vi "day 19 task 1.vi"   [LabVIEW 2019]
uses:
  day 19/robot quantity at time--cluster.ctl
  day 19/supplies--cluster.ctl
  day 19/blueprint--cluster.ctl
types:
  T1 = typedef "supplies--cluster.ctl" = cluster{"ore":i32, "clay":i32, "obsidian":i32, "geode":i32}
  T2 = typedef "robot quantity at time--cluster.ctl" = cluster{"no. ore robots":i32, "no. clay robots":i32, "no. obsidian robots":i32, "no. geode robots":i32, "time elapsed":i32}
  T3 = typedef "blueprint--cluster.ctl" = cluster{"blueprint no.":i32, "cost of ore robot (ore)":i32, "cost of clay robot (ore)":i32, "cost of obsidian robot (ore)":i32, "cost of obsidian robot (clay)":i32, "cost of geode robot (ore)":i32, "cost of geode robot (obsidian)":i32}
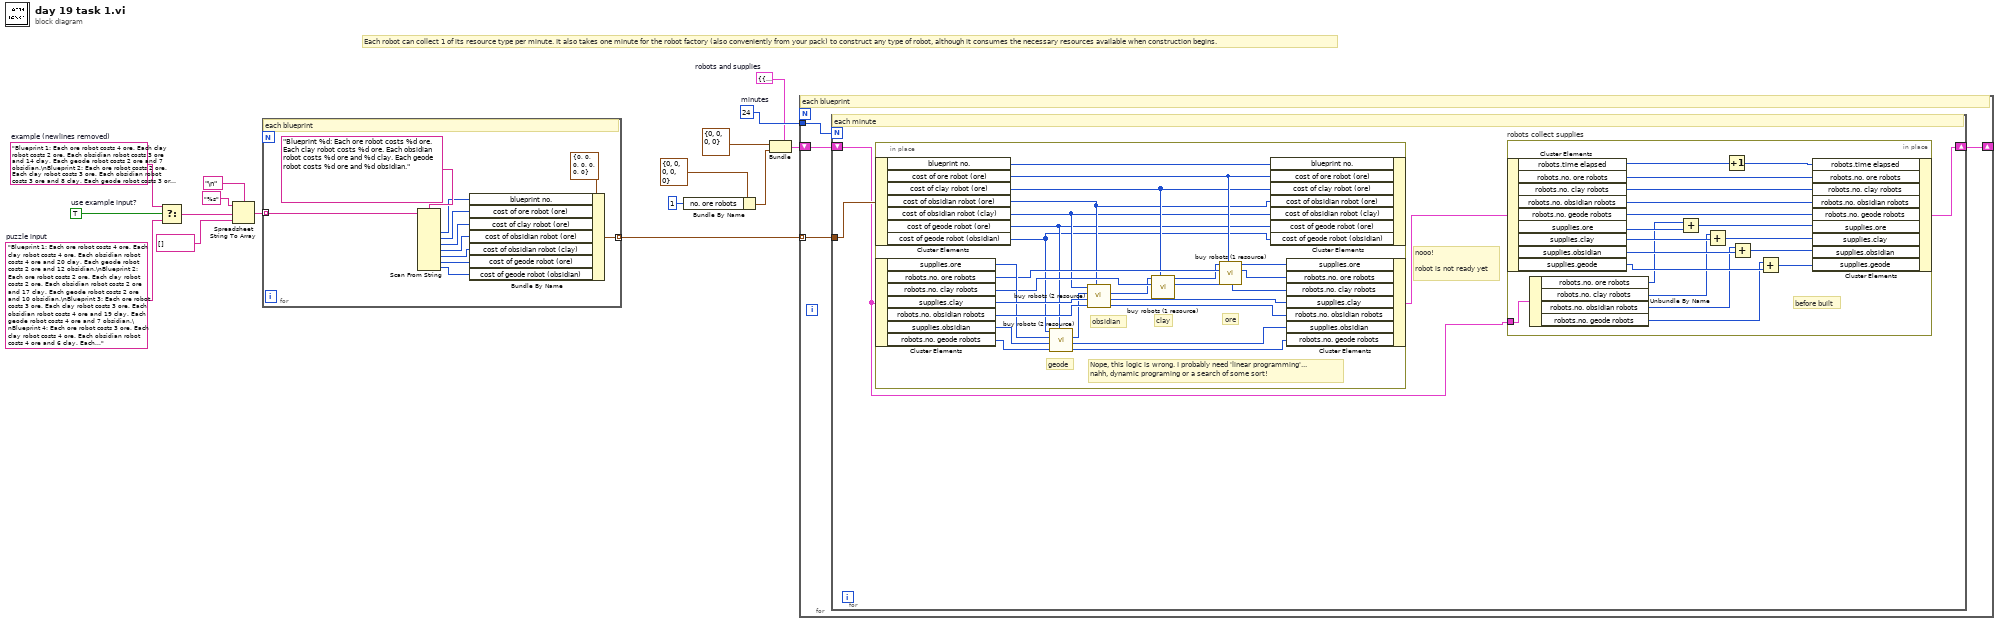
[diagram p0: block diagram]
diagram:
  w1 = cluster{"supplies":T1, "robots":T2} {"supplies"={"ore"=0, "clay"=0, "obsidian"=0, "geode"=0}, "robots"={"no. ore robots"=0, "no. clay robots"=0, "no. obsidian robots"=0, "no. geode robots"=0, "time elapsed"=0}}  # robots and supplies
  w3 = 24  # minutes
  w10 = TRUE  # use example input?
  w11 = "Blueprint 1: Each ore robot costs 4 ore. Each clay robot costs 4 ore. Each obsidian robot costs 4 ore and 20 clay. Each geode robot costs 2 ore and 12 obsidian.\nBlueprint 2: Each ore robot costs 2 ore. Each clay robot costs 2 ore. Each obsidian robot costs 2 ore and 17 clay. Each geode robot costs 2 ore and 10 obsidian.\nBlueprint 3: Each ore robot costs 3 ore. Each clay robot costs 3 ore. Each obsidian robot costs 4 ore and 19 clay. Each geode robot costs 4 ore and 7 obsidian.\nBlueprint 4: Each ore robot costs 3 ore. Each clay robot costs 4 ore. Each obsidian robot costs 4 ore and 6 clay. Each geode robot costs 2 ore and 20 obsidian.\nBlueprint 5: Each ore robot costs 2 ore. Each clay robot costs 4 ore. Each obsidian robot costs 4 ore and 19 clay. Each geode robot costs 2 ore and 18 obsidian.\nBlueprint 6: Each ore robot costs 4 ore. Each clay robot costs 4 ore. Each obsidian robot costs 3 ore and 14 clay. Each geode robot costs 4 ore and 15 obsidian.\nBlueprint 7: Each ore robot costs 3 ore. Each clay robot costs 4 ore. Each obsidian robot costs 3 ore and 15 clay. Each geode robot costs 3 ore and 20 obsidian.\nBlueprint 8: Each ore robot costs 2 ore. Each clay robot costs 4 ore. Each obsidian robot costs 2 ore and 20 clay. Each geode robot costs 3 ore and 15 obsidian.\nBlueprint 9: Each ore robot costs 2 ore. Each clay robot costs 2 ore. Each obsidian robot costs 2 ore and 20 clay. Each geode robot costs 2 ore and 14 obsidian.\nBlueprint 10: Each ore robot costs 4 ore. Each clay robot costs 4 ore. Each obsidian robot costs 4 ore and 5 clay. Each geode robot costs 3 ore and 7 obsidian.\nBlueprint 11: Each ore robot costs 4 ore. Each clay robot costs 3 ore. Each obsidian robot costs 4 ore and 11 clay. Each geode robot costs 3 ore and 15 obsidian.\nBlueprint 12: Each ore robot costs 4 ore. Each clay robot costs 4 ore. Each obsidian robot costs 3 ore and 20 clay. Each geode robot costs 2 ore and 10 obsidian.\nBlueprint 13: Each ore robot costs 4 ore. Each clay robot costs 4 ore. Each obsidian robot costs 4 ore and 7 clay. Each geode robot costs 4 ore and 17 obsidian.\nBlueprint 14: Each ore robot costs 2 ore. Each clay robot costs 4 ore. Each obsidian robot costs 4 ore and 20 clay. Each geode robot costs 3 ore and 14 obsidian.\nBlueprint 15: Each ore robot costs 4 ore. Each clay robot costs 4 ore. Each obsidian robot costs 2 ore and 17 clay. Each geode robot costs 3 ore and 11 obsidian.\nBlueprint 16: Each ore robot costs 4 ore. Each clay robot costs 3 ore. Each obsidian robot costs 2 ore and 14 clay. Each geode robot costs 4 ore and 11 obsidian.\nBlueprint 17: Each ore robot costs 4 ore. Each clay robot costs 3 ore. Each obsidian robot costs 4 ore and 15 clay. Each geode robot costs 4 ore and 9 obsidian.\nBlueprint 18: Each ore robot costs 3 ore. Each clay robot costs 3 ore. Each obsidian robot costs 3 ore and 19 clay. Each geode robot costs 3 ore and 17 obsidian.\nBlueprint 19: Each ore robot costs 4 ore. Each clay robot costs 3 ore. Each obsidian robot costs 2 ore and 20 clay. Each geode robot costs 2 ore and 9 obsidian.\nBlueprint 20: Each ore robot costs 3 ore. Each clay robot costs 4 ore. Each obsidian robot costs 2 ore and 11 clay. Each geode robot costs 2 ore and 10 obsidian.\nBlueprint 21: Each ore robot costs 4 ore. Each clay robot costs 4 ore. Each obsidian robot costs 4 ore and 10 clay. Each geode robot costs 2 ore and 7 obsidian.\nBlueprint 22: Each ore robot costs 4 ore. Each clay robot costs 4 ore. Each obsidian robot costs 3 ore and 6 clay. Each geode robot costs 2 ore and 14 obsidian.\nBlueprint 23: Each ore robot costs 4 ore. Each clay robot costs 4 ore. Each obsidian robot costs 4 ore and 15 clay. Each geode robot costs 3 ore and 8 obsidian.\nBlueprint 24: Each ore robot costs 4 ore. Each clay robot costs 4 ore. Each obsidian robot costs 4 ore and 8 clay. Each geode robot costs 3 ore and 19 obsidian.\nBlueprint 25: Each ore robot costs 2 ore. Each clay robot costs 3 ore. Each obsidian robot costs 3 ore and 9 clay. Each geode robot costs 3 ore and 9 obsidian.\nBlueprint 26: Each ore robot costs 3 ore. Each clay robot costs 3 ore. Each obsidian robot costs 2 ore and 20 clay. Each geode robot costs 2 ore and 20 obsidian.\nBlueprint 27: Each ore robot costs 4 ore. Each clay robot costs 4 ore. Each obsidian robot costs 3 ore and 10 clay. Each geode robot costs 2 ore and 14 obsidian.\nBlueprint 28: Each ore robot costs 2 ore. Each clay robot costs 4 ore. Each obsidian robot costs 3 ore and 19 clay. Each geode robot costs 4 ore and 8 obsidian.\nBlueprint 29: Each ore robot costs 4 ore. Each clay robot costs 4 ore. Each obsidian robot costs 2 ore and 9 clay. Each geode robot costs 3 ore and 19 obsidian.\nBlueprint 30: Each ore robot costs 4 ore. Each clay robot costs 3 ore. Each obsidian robot costs 2 ore and 13 clay. Each geode robot costs 2 ore and 10 obsidian."  # puzzle input
  w12 = "Blueprint 1: Each ore robot costs 4 ore. Each clay robot costs 2 ore. Each obsidian robot costs 3 ore and 14 clay. Each geode robot costs 2 ore and 7 obsidian.\nBlueprint 2: Each ore robot costs 2 ore. Each clay robot costs 3 ore. Each obsidian robot costs 3 ore and 8 clay. Each geode robot costs 3 ore and 12 obsidian."  # example (newlines removed)
  # "Each robot can collect 1 of its resource type per minute. It also takes one minute for the robot factory (also conveniently from your pack) to construct any type of robot, although it consumes the necessary resources available when construction begins."
  n1 = Select(t=w12, s=w10, f=w11) -> (s? t:f=w9:string)
  n2 = Spreadsheet String To Array(delimiter (Tab)="\n", format string="%s", spreadsheet string=w9, array type (2D Dbl)=string[] []) -> (array=w13:string[])
  n3 = for {
    tunnel: w13 -> [w27] mode=indexing
    tunnel: [w17] -> w6 mode=indexing
    # "each blueprint"
    n4 = Scan From String(format string="Blueprint %d: Each ore robot costs %d ore. Each clay robot costs %d ore. Each obsidian robot costs %d ore and %d clay. Each geode robot costs %d ore and %d obsidian.", input string=w27) -> (output 1=w24:i32, output 2=w23:i32, output 3=w22:i32, output 4=w21:i32, output 5=w20:i32, output 6=w19:i32, output 7=w18:i32)  [unwired: 9 in, 3 out]
    n5 = Bundle By Name(cluster=T3 {"blueprint no."=0, "cost of ore robot (ore)"=0, "cost of clay robot (ore)"=0, "cost of obsidian robot (ore)"=0, "cost of obsidian robot (clay)"=0, "cost of geode robot (ore)"=0, "cost of geode robot (obsidian)"=0}, "blueprint no."=w24, "cost of ore robot (ore)"=w23, "cost of clay robot (ore)"=w22, "cost of obsidian robot (ore)"=w21, "cost of obsidian robot (clay)"=w20, "cost of geode robot (ore)"=w19, "cost of geode robot (obsidian)"=w18) -> (w17:T3)
  }
  n6 = Bundle By Name(cluster=T2 {"no. ore robots"=0, "no. clay robots"=0, "no. obsidian robots"=0, "no. geode robots"=0, "time elapsed"=0}, "no. ore robots"=1) -> (w4:T2)
  n7 = Bundle(cluster=w1, "supplies"=T1 {"ore"=0, "clay"=0, "obsidian"=0, "geode"=0}, "robots"=w4) -> (w2:cluster{"supplies":T1, "robots":T2})
  n8 = for {
    tunnel: w6 -> [w30] mode=indexing
    tunnel: w3 -> [w31]
    shift-right: [w28] -> _
    shift-left: w2 -> [w29]
    # "each blueprint"
    n9 = for {
      N: w31 -> [_]
      tunnel: w30 -> [w35]
      shift-right: [w34] -> w28
      shift-left: w29 -> [w33]
      # "nooo!\n\nrobot is not ready yet"
      # "each minute"
      n10 = in-place {
        # "Nope, this logic is wrong. I probably need 'linear programming'...\nnahh, dynamic programing or a search of some sort!"
        # "ore"
        # "clay"
        # "obsidian"
        # "geode"
        n11 = in-place-cluster #1(w35) -> ("blueprint no."=w39:i32, "cost of ore robot (ore)"=w42:i32, "cost of clay robot (ore)"=w41:i32, "cost of obsidian robot (ore)"=w40:i32, "cost of obsidian robot (clay)"=w38:i32, "cost of geode robot (ore)"=w37:i32, "cost of geode robot (obsidian)"=w36:i32)
        n12 = in-place-cluster #2(w33) -> ("supplies.ore"=w56:i32, "robots.no. ore robots"=w46:i32, "robots.no. clay robots"=w50:i32, "supplies.clay"=w59:i32, "robots.no. obsidian robots"=w58:i32, "supplies.obsidian"=w55:i32, "robots.no. geode robots"=w54:i32)
        n13 = call "buy robots (2 resource).vi"("cost of robot (X)"=w37, "no. robots in"=w54, "Y's resource in"=w55, "X's resource in"=w56, "cost of robot (Y)"=w36) -> ("no. robots out"=w53:i32, "Y's resource out"=w51:i32, "X's resource out"=w52:i32)  [unwired: 4 in]
        n14 = call "buy robots (2 resource).vi"("cost of robot (X)"=w40, "no. robots in"=w58, "Y's resource in"=w59, "X's resource in"=w52, "cost of robot (Y)"=w38) -> ("no. robots out"=w57:i32, "Y's resource out"=w49:i32, "X's resource out"=w48:i32)  [unwired: 4 in]
        n15 = call "buy robots (1 resource).vi"("cost of X robot"=w41, "no. X robots in"=w50, "robot's resource in"=w48) -> ("no. X robots out"=w47:i32, "robot's resource out"=w45:i32)  [unwired: 7 in]
        n16 = call "buy robots (1 resource).vi"("cost of X robot"=w42, "no. X robots in"=w46, "robot's resource in"=w45) -> ("no. X robots out"=w43:i32, "robot's resource out"=w44:i32)  [unwired: 7 in]
        n17 = in-place-cluster #1("blueprint no."=w39, "cost of ore robot (ore)"=w42, "cost of clay robot (ore)"=w41, "cost of obsidian robot (ore)"=w40, "cost of obsidian robot (clay)"=w38, "cost of geode robot (ore)"=w37, "cost of geode robot (obsidian)"=w36) -> ()  [unwired: 1 out]
        n18 = in-place-cluster #2("supplies.ore"=w44, "robots.no. ore robots"=w43, "robots.no. clay robots"=w47, "supplies.clay"=w49, "robots.no. obsidian robots"=w57, "supplies.obsidian"=w51, "robots.no. geode robots"=w53) -> (w32:cluster{"supplies":T1, "robots":T2})
      }
      n19 = in-place "robots collect supplies" {
        in-place-border: w33 -> [w68]
        # "before built"
        n20 = in-place-cluster #3(w32) -> ("robots.time elapsed"=w69:i32, "robots.no. ore robots"=w67:i32, "robots.no. clay robots"=w66:i32, "robots.no. obsidian robots"=w65:i32, "robots.no. geode robots"=w64:i32, "supplies.ore"=w78:i32, "supplies.clay"=w77:i32, "supplies.obsidian"=w76:i32, "supplies.geode"=w75:i32)
        n21 = Unbundle By Name(w68) -> ("robots.no. ore robots"=w63:i32, "robots.no. clay robots"=w62:i32, "robots.no. obsidian robots"=w61:i32, "robots.no. geode robots"=w60:i32)
        n22 = Add(x=w63, y=w78) -> (x+y=w71:i32)
        n23 = Add(x=w62, y=w77) -> (x+y=w72:i32)
        n24 = Increment(x=w69) -> (x+1=w70:i32)
        n25 = Add(x=w61, y=w76) -> (x+y=w73:i32)
        n26 = Add(x=w60, y=w75) -> (x+y=w74:i32)
        n27 = in-place-cluster #3("robots.time elapsed"=w70, "robots.no. ore robots"=w67, "robots.no. clay robots"=w66, "robots.no. obsidian robots"=w65, "robots.no. geode robots"=w64, "supplies.ore"=w71, "supplies.clay"=w72, "supplies.obsidian"=w73, "supplies.geode"=w74) -> (w34:cluster{"supplies":T1, "robots":T2})
      }
    }
  }
